vi "Array_compensation_sub.vi"(1 "all rows":dbl[][](array[numeric])=[[0.0, 0.0, 0.0, 0.0, 0.0, 0.0, 0.0, 0.0, 0.0, 0.0, 0.0, 0.0, 0.0, 0.0, 0.0, 0.0, 0.0, 0.0, 0.0, 0.0, 0.0, 0.0, 0.0, 0.0, 0.0, 0.0, 0.0, 0.0, 0.0], [0.0, 0.0, 0.0, 0.0, 0.0, 0.0, 0.0, 0.0, 0.0, 0.0, 0.0, 0.0, 0.0, 0.0, 0.0, 0.0, 0.0, 0.0, 0.0, 0.0, 0.0, 0.0, 0.0, 0.0, 0.0, 0.0, 0.0, 0.0, 0.0], [0.0, 0.0, 0.0, 0.0, 0.0, 0.0, 0.0, 0.0, 0.0, 0.0, 0.0, 0.0, 0.0, 0.0, 0.0, 0.0, 0.0, 0.0, 0.0, 0.0, 0.0, 0.0, 0.0, 0.0, 0.0, 0.0, 0.0, 0.0, 0.0], [0.0, 0.0, 0.0, 0.0, 0.0, 0.0, 0.0, 0.0, 0.0, 0.0, 0.0, 0.0, 0.0, 0.0, 0.0, 0.0, 0.0, 0.0, 0.0, 0.0, 0.0, 0.0, 0.0, 0.0, 0.0, 0.0, 0.0, 0.0, 0.0], [0.0, 0.0, 0.0, 0.0, 0.0, 0.0, 0.0, 0.0, 0.0, 0.0, 0.0, 0.0, 0.0, 0.0, 0.0, 0.2, 0.6235294117647059, 0.9921568627450981, 0.6235294117647059, 0.19607843137254902, 0.0, 0.0, 0.0, 0.0, 0.0, 0.0, 0.0, 0.0, 0.0], [0.0, 0.0, 0.0, 0.0, 0.0, 0.0, 0.0, 0.0, 0.0, 0.0, 0.0, 0.0, 0.0, 0.0, 0.18823529411764706, 0.9333333333333333, 0.9882352941176471, 0.9882352941176471, 0.9882352941176471, 0.9294117647058824, 0.0, 0.0, 0.0, 0.0, 0.0, 0.0, 0.0, 0.0, 0.0], [0.0, 0.0, 0.0, 0.0, 0.0, 0.0, 0.0, 0.0, 0.0, 0.0, 0.0, 0.0, 0.0, 0.21176470588235294, 0.8901960784313725, 0.9921568627450981, 0.9882352941176471, 0.9372549019607843, 0.9137254901960784, 0.9882352941176471, 0.2235294117647059, 0.023529411764705882, 0.0, 0.0, 0.0, 0.0, 0.0, 0.0, 0.0], [0.0, 0.0, 0.0, 0.0, 0.0, 0.0, 0.0, 0.0, 0.0, 0.0, 0.0, 0.0392156862745098, 0.23529411764705882, 0.8784313725490196, 0.9882352941176471, 0.9921568627450981, 0.9882352941176471, 0.792156862745098, 0.32941176470588235, 0.9882352941176471, 0.9921568627450981, 0.47843137254901963, 0.0, 0.0, 0.0, 0.0, 0.0, 0.0, 0.0], [0.0, 0.0, 0.0, 0.0, 0.0, 0.0, 0.0, 0.0, 0.0, 0.0, 0.0, 0.6392156862745098, 0.9882352941176471, 0.9882352941176471, 0.9882352941176471, 0.9921568627450981, 0.9882352941176471, 0.9882352941176471, 0.3764705882352941, 0.7411764705882353, 0.9921568627450981, 0.6549019607843137, 0.0, 0.0, 0.0, 0.0, 0.0, 0.0, 0.0], [0.0, 0.0, 0.0, 0.0, 0.0, 0.0, 0.0, 0.0, 0.0, 0.0, 0.2, 0.9333333333333333, 0.9921568627450981, 0.9921568627450981, 0.7450980392156863, 0.4470588235294118, 0.9921568627450981, 0.8941176470588236, 0.1843137254901961, 0.30980392156862746, 1.0, 0.6588235294117647, 0.0, 0.0, 0.0, 0.0, 0.0, 0.0, 0.0], [0.0, 0.0, 0.0, 0.0, 0.0, 0.0, 0.0, 0.0, 0.0, 0.18823529411764706, 0.9333333333333333, 0.9882352941176471, 0.9882352941176471, 0.7019607843137254, 0.047058823529411764, 0.29411764705882354, 0.4745098039215686, 0.08235294117647059, 0.0, 0.0, 0.9921568627450981, 0.9529411764705882, 0.19607843137254902, 0.0, 0.0, 0.0, 0.0, 0.0, 0.0], [0.0, 0.0, 0.0, 0.0, 0.0, 0.0, 0.0, 0.0, 0.14901960784313725, 0.6470588235294118, 0.9921568627450981, 0.9137254901960784, 0.8156862745098039, 0.32941176470588235, 0.0, 0.0, 0.0, 0.0, 0.0, 0.0, 0.9921568627450981, 0.9882352941176471, 0.6470588235294118, 0.0, 0.0, 0.0, 0.0, 0.0, 0.0], [0.0, 0.0, 0.0, 0.0, 0.0, 0.0, 0.0, 0.027450980392156862, 0.6980392156862745, 0.9882352941176471, 0.9411764705882353, 0.2784313725490196, 0.07450980392156863, 0.10980392156862745, 0.0, 0.0, 0.0, 0.0, 0.0, 0.0, 0.9921568627450981, 0.9882352941176471, 0.7647058823529411, 0.0, 0.0, 0.0, 0.0, 0.0, 0.0], [0.0, 0.0, 0.0, 0.0, 0.0, 0.0, 0.0, 0.2235294117647059, 0.9882352941176471, 0.9882352941176471, 0.24705882352941178, 0.0, 0.0, 0.0, 0.0, 0.0, 0.0, 0.0, 0.0, 0.0, 0.9921568627450981, 0.9882352941176471, 0.7647058823529411, 0.0, 0.0, 0.0, 0.0, 0.0, 0.0], [0.0, 0.0, 0.0, 0.0, 0.0, 0.0, 0.0, 0.7764705882352941, 0.9921568627450981, 0.7450980392156863, 0.0, 0.0, 0.0, 0.0, 0.0, 0.0, 0.0, 0.0, 0.0, 0.0, 1.0, 0.9921568627450981, 0.7686274509803922, 0.0, 0.0, 0.0, 0.0, 0.0, 0.0], [0.0, 0.0, 0.0, 0.0, 0.0, 0.0, 0.2980392156862745, 0.9647058823529412, 0.9882352941176471, 0.4392156862745098, 0.0, 0.0, 0.0, 0.0, 0.0, 0.0, 0.0, 0.0, 0.0, 0.0, 0.9921568627450981, 0.9882352941176471, 0.5803921568627451, 0.0, 0.0, 0.0, 0.0, 0.0, 0.0], [0.0, 0.0, 0.0, 0.0, 0.0, 0.0, 0.3333333333333333, 0.9882352941176471, 0.9019607843137255, 0.09803921568627451, 0.0, 0.0, 0.0, 0.0, 0.0, 0.0, 0.0, 0.0, 0.027450980392156862, 0.5294117647058824, 0.9921568627450981, 0.7294117647058823, 0.047058823529411764, 0.0, 0.0, 0.0, 0.0, 0.0, 0.0], [0.0, 0.0, 0.0, 0.0, 0.0, 0.0, 0.3333333333333333, 0.9882352941176471, 0.8745098039215686, 0.0, 0.0, 0.0, 0.0, 0.0, 0.0, 0.0, 0.0, 0.027450980392156862, 0.5137254901960784, 0.9882352941176471, 0.8823529411764706, 0.2784313725490196, 0.0, 0.0, 0.0, 0.0, 0.0, 0.0, 0.0], [0.0, 0.0, 0.0, 0.0, 0.0, 0.0, 0.3333333333333333, 0.9882352941176471, 0.5686274509803921, 0.0, 0.0, 0.0, 0.0, 0.0, 0.0, 0.0, 0.18823529411764706, 0.6470588235294118, 0.9882352941176471, 0.6784313725490196, 0.0, 0.0, 0.0, 0.0, 0.0, 0.0, 0.0, 0.0, 0.0], [0.0, 0.0, 0.0, 0.0, 0.0, 0.0, 0.33725490196078434, 0.9921568627450981, 0.8823529411764706, 0.0, 0.0, 0.0, 0.0, 0.0, 0.0, 0.4470588235294118, 0.9333333333333333, 0.9921568627450981, 0.6352941176470588, 0.0, 0.0, 0.0, 0.0, 0.0, 0.0, 0.0, 0.0, 0.0, 0.0], [0.0, 0.0, 0.0, 0.0, 0.0, 0.0, 0.3333333333333333, 0.9882352941176471, 0.9764705882352941, 0.5725490196078431, 0.18823529411764706, 0.11372549019607843, 0.3333333333333333, 0.6980392156862745, 0.8823529411764706, 0.9921568627450981, 0.8745098039215686, 0.6549019607843137, 0.2196078431372549, 0.0, 0.0, 0.0, 0.0, 0.0, 0.0, 0.0, 0.0, 0.0, 0.0], [0.0, 0.0, 0.0, 0.0, 0.0, 0.0, 0.3333333333333333, 0.9882352941176471, 0.9882352941176471, 0.9882352941176471, 0.8980392156862745, 0.8431372549019608, 0.9882352941176471, 0.9882352941176471, 0.9882352941176471, 0.7686274509803922, 0.5098039215686274, 0.0, 0.0, 0.0, 0.0, 0.0, 0.0, 0.0, 0.0, 0.0, 0.0, 0.0, 0.0], [0.0, 0.0, 0.0, 0.0, 0.0, 0.0, 0.10980392156862745, 0.7803921568627451, 0.9882352941176471, 0.9882352941176471, 0.9921568627450981, 0.9882352941176471, 0.9882352941176471, 0.9137254901960784, 0.5686274509803921, 0.0, 0.0, 0.0, 0.0, 0.0, 0.0, 0.0, 0.0, 0.0, 0.0, 0.0, 0.0, 0.0, 0.0], [0.0, 0.0, 0.0, 0.0, 0.0, 0.0, 0.0, 0.09803921568627451, 0.5019607843137255, 0.9882352941176471, 0.9921568627450981, 0.9882352941176471, 0.5529411764705883, 0.1450980392156863, 0.0, 0.0, 0.0, 0.0, 0.0, 0.0, 0.0, 0.0, 0.0, 0.0, 0.0, 0.0, 0.0, 0.0, 0.0], [0.0, 0.0, 0.0, 0.0, 0.0, 0.0, 0.0, 0.0, 0.0, 0.0, 0.0, 0.0, 0.0, 0.0, 0.0, 0.0, 0.0, 0.0, 0.0, 0.0, 0.0, 0.0, 0.0, 0.0, 0.0, 0.0, 0.0, 0.0, 0.0], [0.0, 0.0, 0.0, 0.0, 0.0, 0.0, 0.0, 0.0, 0.0, 0.0, 0.0, 0.0, 0.0, 0.0, 0.0, 0.0, 0.0, 0.0, 0.0, 0.0, 0.0, 0.0, 0.0, 0.0, 0.0, 0.0, 0.0, 0.0, 0.0], [0.0, 0.0, 0.0, 0.0, 0.0, 0.0, 0.0, 0.0, 0.0, 0.0, 0.0, 0.0, 0.0, 0.0, 0.0, 0.0, 0.0, 0.0, 0.0, 0.0, 0.0, 0.0, 0.0, 0.0, 0.0, 0.0, 0.0, 0.0, 0.0], [0.0, 0.0, 0.0, 0.0, 0.0, 0.0, 0.0, 0.0, 0.0, 0.0, 0.0, 0.0, 0.0, 0.0, 0.0, 0.0, 0.0, 0.0, 0.0, 0.0, 0.0, 0.0, 0.0, 0.0, 0.0, 0.0, 0.0, 0.0, 0.0]]) -> (0 "CompensatedArray":dbl[][](array[numeric]))   [LabVIEW 2021]
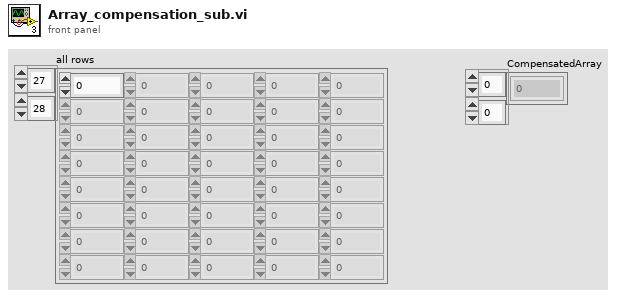
[diagram p1: front panel]
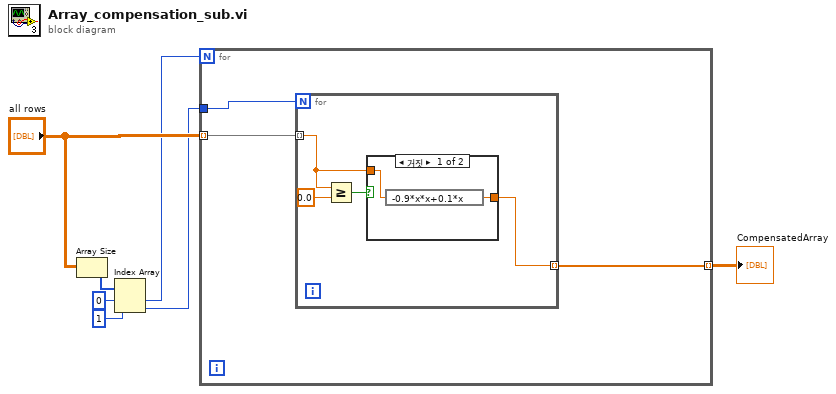
[diagram p0: block diagram]
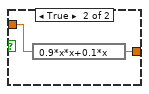
[diagram p2: hidden frame]
diagram:
  n1 = Array Size(array="all rows") -> (size(s)=w6:i32[])
  n2 = Index Array(array=w6, index #1=0 ("인덱스"), index #2=1 ("인덱스")) -> (element #1=w3:i32, element #2=w2:i32)
  n3 = for {
    N: w3 -> [_]
    tunnel: "all rows" -> [w10] mode=indexing
    tunnel: w2 -> [w9]
    tunnel: [w8] -> w1 mode=indexing
    n4 = for {
      N: w9 -> [_]
      tunnel: w10 -> [w12] mode=indexing
      tunnel: [w11] -> w8 mode=indexing
      n5 = Greater Or Equal?(x=w12, y=0.0) -> (x >= y?=w14:bool)
      n6 = case shown="거짓" w14 {
        tunnel: w12 -> [w16 w18]
        tunnel: [w15 w17] -> w11
        frame False {
          n7 = expression code="-0.9*x*x+0.1*x"(w16) -> (w15:dbl)
        }
        frame True {
          n8 = expression code="0.9*x*x+0.1*x"(w18) -> (w17:dbl)
        }
      }
    }
  }
  "CompensatedArray" <- w1
